vi "TruncatedSVD.vi"(8 "error in":errorcluster) -> (0 "error out":errorcluster, 3 "out":refnum<class "TruncatedSVD.lvclass">)   [LabVIEW 2020]
doc: "Dimensionality reduction using truncated SVD (aka LSA).\n\n This transformer performs linear dimensionality reduction by means of\n truncated singular value decomposition (SVD). Contrary to PCA, this\n estimator does not center the data before computing the singular value\n decomposition. This means it can work with sparse matrices\n efficiently.\n\n In particular, truncated SVD works on term count/tf-idf matrices as\n returned by the vectorizers in :mod:`sklearn.feature_extraction.text`. In\n that context, it is known as latent semantic analysis (LSA).\n\n This estimator supports two algorithms: a fast randomized SVD solver, and\n a \"naive\" algorithm that uses ARPACK as an eigensolver on `X * X.T` or\n `X.T * X`, whichever is more efficient.\n\n Read more in the :ref:`User Guide <LSA>`.\n\n Parameters\n ----------\n n_components : int, default=2\n Desired dimensionality of output data.\n Must be strictly less than the number of features.\n The default value is useful for visualisation. For LSA, a value of\n 100 is recommended.\n\n algorithm : {'arpack', 'randomized'}, default='randomized'\n SVD solver to use. Either \"arpack\" for the ARPACK wrapper in SciPy\n (scipy.sparse.linalg.svds), or \"randomized\" for the randomized\n algorithm due to Halko (2009).\n\n n_iter : int, default=5\n Number of iterations for randomized SVD solver. Not used by ARPACK. The\n default is larger than the default in\n :func:`~sklearn.utils.extmath.randomized_svd` to handle sparse\n matrices that may have large slowly decaying spectrum.\n\n random_state : int, RandomState instance or None, default=None\n Used during randomized svd. Pass an int for reproducible results across\n multiple function calls.\n See :term:`Glossary <random_state>`.\n\n tol : float, default=0.\n Tolerance for ARPACK. 0 means machine precision. Ignored by randomized\n SVD solver.\n\n Attributes\n ----------\n components_ : ndarray of shape (n_components, n_features)\n\n explained_variance_ : ndarray of shape (n_components,)\n The variance of the training samples transformed by a projection to\n each component.\n\n explained_variance_ratio_ : ndarray of shape (n_components,)\n Percentage of variance explained by each of the selected components.\n\n singular_values_ : ndarray od shape (n_components,)\n The singular values corresponding to each of the selected components.\n The singular values are equal to the 2-norms of the ``n_components``\n variables in the lower-dimensional space.\n\n \nAvailable methods:\nFit\nFit Transform\nTransform\nGet Attributes\nGet Params\nSet Params"
uses:
  TruncatedSVD.lvclass
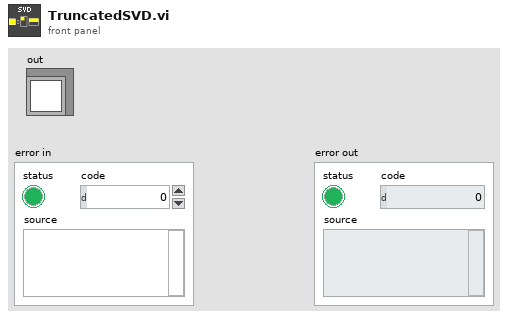
[diagram p1: front panel]
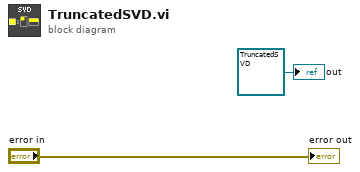
[diagram p0: block diagram]
diagram:
  "out" <- refnum<class "TruncatedSVD.lvclass"> refnum ("model")
  "error out" <- "error in"
